vi "Waka manual control.vi"() -> ()   [LabVIEW 2024]
uses:
  ZeroJet Test Systems/Production Data/Production Data.lvlib
  <instrlib>/KDI Digital Instrumentation/API_for_PCAN_BASIC_FD/TPCANBaudrate.ctl
  <instrlib>/KDI Digital Instrumentation/API_for_PCAN_BASIC_FD/TPCANHandle.ctl
  ZeroJet Test Systems/Production Data/TestStand Results/MEASUREMENT power spectrum.vi
  <vilib>/Utility/error.llb/DialogType.ctl
  <userlib>/ZeroJet/IT6000C/IT6000C production.lvlib
  <vilib>/platform/TimedLoop/XDataNode/XDataNode.xnode
  <vilib>/Platform/TimedLoop/XDataNode/nitl_modes.ctl
  <vilib>/Platform/TimedLoop/XDataNode/XDNodeRunTimeDep.lvlib
  <vilib>/Platform/TimedLoop/XDataNode/wakeup.ctl
  <vilib>/Platform/TimedLoop/XDataNode/timing_clust.ctl
  ZeroJet Test Systems/Production Data/TestStand Results/MEASUREMENT float.vi
  ZeroJet Test Systems/Instruments/PCAN/PCan_Xnet.lvlib
  <instrlib>/IT6000C/IT6000C.lvlib
  <vilib>/Utility/sysdir.llb/System Directory Type.ctl
  Helper/Key CAN statistics.ctl
panel:
  in  "stop":bool
  out "Main selector":enum32{"Power supply Setup", "CAN Setup", "Run"}(tab)
  in  "IT6000C instrument address":refnum<visa-resource-name>="USB0::0x2EC7::0x6000::804050011767650001::INSTR"
  in  "Voltage rise time":dbl=5.0 format="%#_13gs"
  in  "Power supply watchdog time":dbl=2.0 min=0.0 max=10.0 step=0.1 format="%#_13gs"
  in  "Button - Connect power supply":bool
  in  "Button - Don't use power supply":bool
  out "LED - Supply connected":bool
  out "Connection response":string
  in  "Button - Power supply next":bool
  in  "Button - Power supply next":bool
  out "LED - Setting up CAN":bool
  out "CAN Status":string
  in  "Vibration capture time (s)":dbl=60.0
  in  "Batch Serial Number":string="RevC Pilot Run"
  in  "Part Number":string="RevC Jet Pump"
  in  "Serial Number":string
  in  "Button - Reset hour counter":bool
  out "Left spectrum channel":cluster{"f0":dbl, "df":dbl, "magnitude":dbl[]}(graph)
  out "Right spectrum channel":cluster{"f0":dbl, "df":dbl, "magnitude":dbl[]}(graph)
  in  "Run tab data":enum32{"Key Data", "All can data", "Errors"}(tab)
  out "Supply wattage output":dbl format="%.2g"
  in  "Current setpoint":dbl(knob) min=0.0 scale=0.06..300.0
  in  "Supply output state":bool
  out "Supply voltage output":dbl format="%.2g"
  out "Supply current output":dbl format="%.2g"
  in  "Voltage setpoint":dbl(knob) min=0.0 scale=0.06..60.0
  out "Key statistics":T1
  out "Signal map":map{string, dbl}(c390)
  out "Error and warning map":map{string, i8}(c390)
  out "Can data write loop":errorcluster
  out "Power supply update loop":errorcluster
  out "Setup loop":errorcluster
  out "Spectrum loop":errorcluster
  # "Power supply setup"
  # "1. Click in this box and select the instrument address for the power supply\n\n\n\n2. Choose the voltage rise time and the watchdog time\n    - Default: 5s votlage rise time\n    - Default: 2s power supply watchdog time\nYou will likely not need to modify these numbers\n\n\n3. Click on connect or don't use power supply\n    - If you are using a battery, then select don't use"
  # "UUT Details"
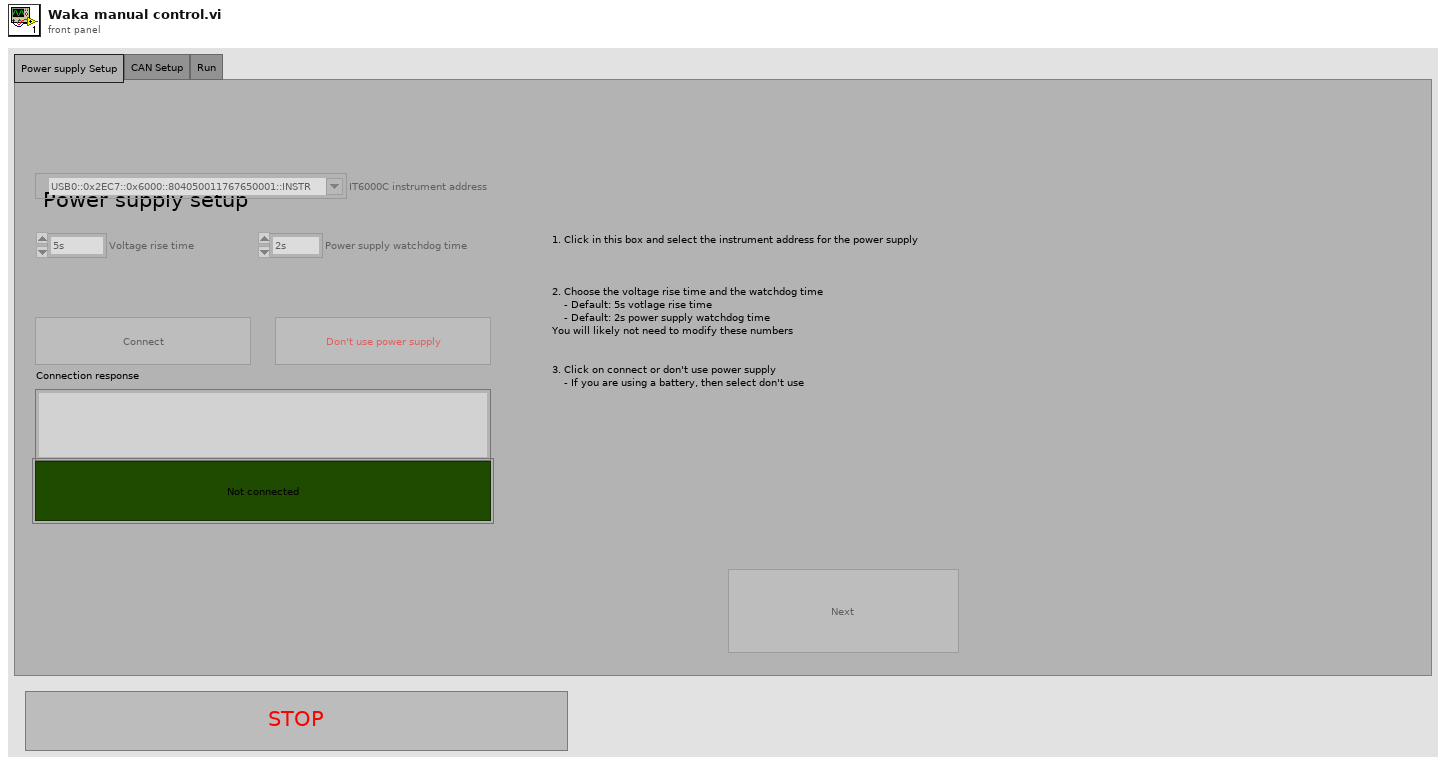
[diagram p1: front panel]
types:
  T1 = typedef "Key CAN statistics.ctl" = cluster{"Drive voltage ":dbl, "High current volt drop":dbl, "High current series resistance":dbl, "Drive phase amps":dbl, "Torque request":dbl, "Motor temp":dbl, "GPS Status":dbl, "RPM":dbl, "Capacitor temp":dbl, "MCM ID":dbl, "MCM Version":string}
  T2 = enum8{"Enabled", "Disabled", "Disabled and Grayed Out"}
  T3 = typedef "TPCANBaudrate.ctl" = enum16{"PCAN_BAUD_1M 0x0014", "PCAN_BAUD_800K 0x0016", "PCAN_BAUD_500K 0x001C", "PCAN_BAUD_250K 0x011C", "PCAN_BAUD_125K 0x031C", "PCAN_BAUD_100K 0x432F", "PCAN_BAUD_95K 0xC34E", "PCAN_BAUD_83K 0x852B", "PCAN_BAUD_50K 0x472F", "PCAN_BAUD_47K 0x1414", "PCAN_BAUD_33K 0x8B2F", "PCAN_BAUD_20K 0x532F", "PCAN_BAUD_10K 0x672F", "PCAN_BAUD_5K 0x7F7F", "User Baudrate"}
  T4 = typedef "TPCANHandle.ctl" = enum16{"PCAN_NONEBUS  0x000", "PCAN_ISABUS1  0x21", "PCAN_ISABUS2  0x22", "PCAN_ISABUS3  0x23", "PCAN_ISABUS4  0x24", "PCAN_ISABUS5  0x25", "PCAN_ISABUS6  0x26", "PCAN_ISABUS7  0x27", "PCAN_ISABUS8  0x28", "PCAN_DNGBUS1  0x31", "PCAN_PCIBUS1  0x41", "PCAN_PCIBUS1  0x42", "PCAN_PCIBUS1  0x43", "PCAN_PCIBUS1  0x44", "PCAN_PCIBUS1  0x45", "PCAN_PCIBUS1  0x46", "PCAN_PCIBUS1  0x47", "PCAN_PCIBUS1  0x48", "PCAN_PCIBUS1  0x409", "PCAN_PCIBUS1  0x40A", "PCAN_PCIBUS1  0x40B", "PCAN_PCIBUS1  0x40C", "PCAN_PCIBUS1  0x40D", "PCAN_PCIBUS1  0x40E", "PCAN_PCIBUS1  0x40F", "PCAN_PCIBUS1  0x410", "PCAN_USBBUS1  0x51", "PCAN_USBBUS2  0x52", "PCAN_USBBUS3  0x53", "PCAN_USBBUS4  0x54", "PCAN_USBBUS5  0x55", "PCAN_USBBUS6  0x56", "PCAN_USBBUS7  0x57", "PCAN_USBBUS8  0x58", "PCAN_USBBUS9  0x509", "PCAN_USBBUS10  0x50A", "PCAN_USBBUS11  0x50B", "PCAN_USBBUS12  0x50C", "PCAN_USBBUS13  0x50D", "PCAN_USBBUS14  0x50E", "PCAN_USBBUS15  0x50F", "PCAN_USBBUS16  0x510", "PCAN_PCCBUS1  0x61", "PCAN_PCCBUS2  0x62", "PCAN_LANBUS1  0x801", "PCAN_LANBUS2  0x802", "PCAN_LANBUS3  0x803", "PCAN_LANBUS4  0x804", "PCAN_LANBUS5  0x805", "PCAN_LANBUS6  0x806", "PCAN_LANBUS7  0x807", "PCAN_LANBUS8  0x808", "PCAN_LANBUS9  0x809", "PCAN_LANBUS10  0x80A", "PCAN_LANBUS11  0x80B", "PCAN_LANBUS12  0x80C", "PCAN_LANBUS13  0x80D", "PCAN_LANBUS14  0x80E", "PCAN_LANBUS15  0x80F", "PCAN_LANBUS16  0x810"}
  T5 = typedef "DialogType.ctl" = u16
  T6 = typedef "NI_Database_API.lvlib/Conn ObjectReference.ctl" = refnum<k1>
  T7 = typedef "System Directory Type.ctl" = i32
  T8 = enum16{"open", "open or create", "create or replace", "create", "open (read-only)"}
  T9 = typedef "XDNodeRunTimeDep.lvlib/timing_clust.ctl" = cluster{"Expected End [f-1]":u64, "Actual End [f-1]":u64, "Finished Late? [f-1]":bool, "Expected End [i-1]":u64, "Actual End [i-1]":u64, "Finished Late? [i-1]":bool, "Expected Start [i]":u64, "Actual Start [i]":u64, "Expected Start [f]":u64, "Actual Start [f]":u64, "Source Name":string, "Structure Name":string, "Period":i64, "Deadline":i64, "Offset":i64, "Start":i64, "Priority":i32, "Timeout":i32, "Mode":T10, "Wakeup Reason":T11, "Error":errorcluster, "Source Type":string, "Secondary Source Type":string, "Global End Time":u64, "Global Start Time":u64, "Frame Duration":u64, "Iteration Duration":u64, "Assigned CPU":i32, "I/O Scan Engine Mode":u32}
  T10 = typedef "XDNodeRunTimeDep.lvlib/nitl_modes.ctl" = enum32{"No Change", "Process missed periods, maintain original phase", "Discard missed periods, maintain original phase", "Process missed periods, ignore original phase", "Discard missed periods, ignore original phase"}
  T11 = typedef "XDNodeRunTimeDep.lvlib/wakeup.ctl" = enum32{"Normal", "Aborted", "Asynchronous wakeup", "Timing source error", "Timed loop error", "Timeout"}
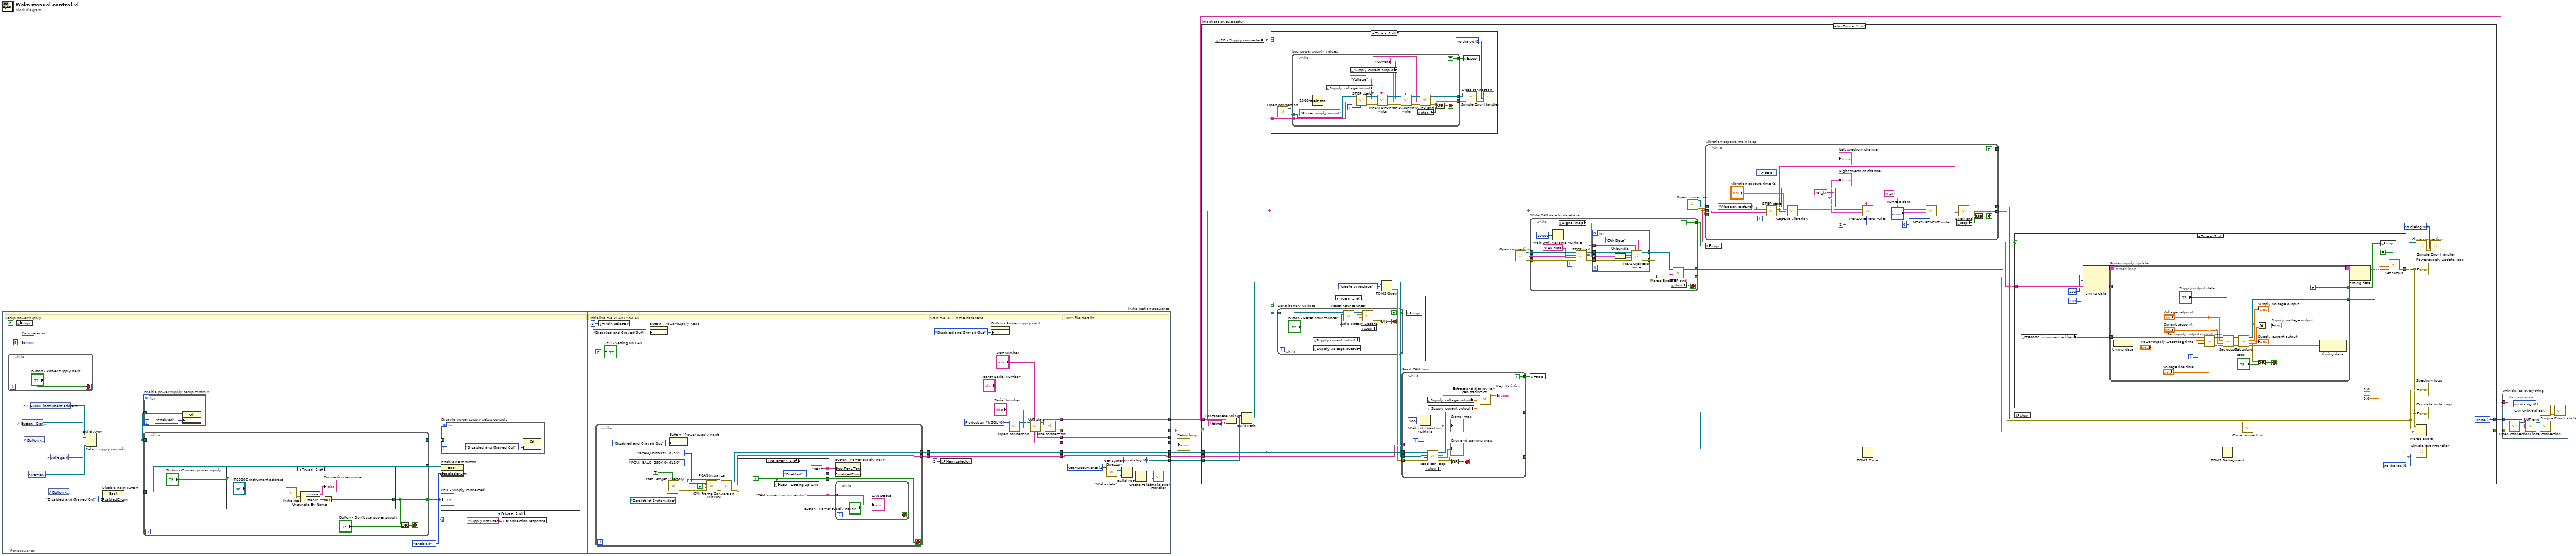
[diagram p0: block diagram]
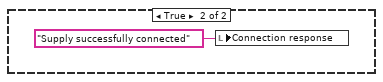
[diagram p2: hidden frame]
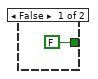
[diagram p3: hidden frame]
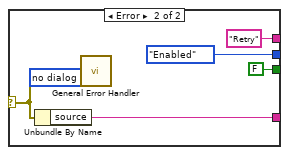
[diagram p4: hidden frame]
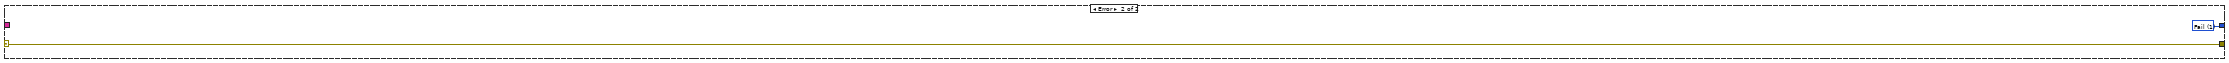
[diagram p8: hidden frame]
diagram:
  n1 = flat-sequence "Initialization sequence" {
    tunnel: [w52] -> w13
    tunnel: [w51] -> w12
    tunnel: w13 -> [w85]
    tunnel: w12 -> [w84]
    tunnel: [w98] -> w9
    tunnel: [w97] -> w8
    tunnel: [w96] -> w7
    tunnel: [w88] -> w6
    tunnel: [w85] -> w5
    tunnel: [w84] -> w4
    tunnel: [w107] -> w10
    tunnel: [w108] -> w11
    tunnel: [w101] -> w2
    tunnel: [w109] -> _
    tunnel: [w110] -> _
    tunnel: [w111] -> w15
    tunnel: w9 -> [w111]
    tunnel: w8 -> [w110]
    tunnel: w7 -> [w109]
    tunnel: w6 -> [w101]
    tunnel: w5 -> [w108]
    tunnel: w4 -> [w107]
    tunnel: [w103] -> w3
    frame #0 {
      # "Setup power supply"
      n2 = while {
        stop <- "Button - Power supply next" stop-if-true
      }
      n3 = local write "stop"(FALSE ("Release all channels first")) -> ()
      n4 = control-ref of="Button - Don't use power supply"() -> (w29:refnum<vi>)
      n5 = control-ref of="Button - Connect power supply"() -> (w28:refnum<vi>)
      n6 = control-ref of="Power supply watchdog time"() -> (w26:refnum<vi>)
      n7 = control-ref of="IT6000C instrument address"() -> (w30:refnum<vi>)
      n8 = control-ref of="Button - Power supply next"() -> (w22:refnum<vi>)
      n9 = control-ref of="Voltage rise time"() -> (w27:refnum<vi>)
      n10 = Build Array "Select supply controls"(w30, w29, w28, w27, w26) -> (w24:refnum<vi>[])
      n11 = property on="Disable next button" class="Bool"(reference=w22, "DisabledEnum"=T2."Disabled and Grayed Out" ("Disabled")) -> (reference out=w19:refnum<vi>)  [unwired: 1 in, 1 out]
      n12 = for "Enable power supply setup controls" {
        tunnel: w24 -> [w34] mode=indexing
        n13 = property class="Ctl"(reference=w34, "DisabledEnum"=T2."Enabled" ("Disabled")) -> ()  [unwired: 1 in, 2 out]
      }
      n14 = while {
        tunnel: [w40] -> w17
        tunnel: [w39] -> w25
        tunnel: w24 -> [w39]
        tunnel: [w38] -> w20
        tunnel: w19 -> [w38]
        stop <- w41 stop-if-true
        n15 = case shown="True" "Button - Connect power supply" {
          tunnel: [FALSE w46] -> w40
          frame False {
          }
          frame True {
            n16 = call <instrlib>:"Initialize.vi"("VISA resource name"="IT6000C instrument address") -> ("error out"=w48:errorcluster)  [unwired: 9 in, 1 out]
            n17 = Unbundle By Name(w48) -> ("source"=→"Connection response":string, "status"=w47:bool)
            n18 = Not(x=w47) -> (.not. x?=w46:bool)
          }
        }
        n19 = Or(x=w40, y="Button - Don't use power supply") -> (x .or. y?=w41:bool)
      }
      "LED - Supply connected" <- w17
      n20 = for "Disable power supply setup controls" {
        tunnel: w25 -> [w32] mode=indexing
        n21 = property class="Ctl"(reference=w32, "DisabledEnum"=T2."Disabled and Grayed Out" ("Disabled")) -> ()  [unwired: 1 in, 2 out]
      }
      n22 = property on="Enable next button" class="Bool"(reference=w20, "DisabledEnum"=T2."Enabled" ("Disabled")) -> ()  [unwired: 1 in, 2 out]
      n23 = case "Update connection response" shown="False" w17 {
        frame False {
          n24 = local write "Connection response"("Supply not used" ("Connection response")) -> ()
        }
        frame True {
          n25 = local write "Connection response"("Supply successfully connected" ("Connection response")) -> ()
        }
      }
      "Main selector" <- 0
    }
    frame #1 {
      # "Initialise the PCAN USB-CAN"
      n26 = while {
        tunnel: [w66] -> w51
        tunnel: [w65] -> w52
        stop <- w57 stop-if-true
        n27 = call "Get ZeroJet Directory.vi"("Expect file to be present"=TRUE, "Data directory subpath"=path "ZeroJet Jet System.dbc") -> ("error out"=w62:errorcluster, "appended path"=w63:path)  [unwired: 7 in, 1 out]
        n28 = property on="Button - Power supply next" class="Bool"("DisabledEnum"=T2."Disabled and Grayed Out" ("Disabled")) -> ()  [unwired: 2 in, 2 out]
        n29 = call "PCAN Initialize.vi"("error in"=w62, "Release all channels first"=TRUE, "TPCANBaudrate"=TPCANBaudrate."PCAN_BAUD_250K 0x011C", "TPCANHandle"=TPCANHandle."PCAN_USBBUS1  0x51") -> ("error out"=w67:errorcluster)  [unwired: 6 in, 1 out]
        n30 = call "CAN Frame Conversion - Init DBC.vi"("error in (no error)"=w67, "DBC Path"=w63) -> ("error out"=w61:errorcluster, "Signals For Conversion"=w66:string[], "Frame Signal Conversion out"=w65:refnum<class "Frame Signal Conversion.lvclass">)  [unwired: 7 in]
        n31 = case shown="No Error" w61 {
          selector: w61 -> [_ w76]
          tunnel: ["Next" ("Boolean Text.Text") "Retry" ("Boolean Text.Text")] -> w59
          tunnel: [T2."Enabled" ("Disabled") T2."Enabled" ("Disabled")] -> w58
          tunnel: ["CAN connection successful" ("source") w78] -> w56
          tunnel: [w71 FALSE ("LED - Setting up CAN")] -> w57
          frame No Error {
            w71 = TRUE ("LED - Setting up CAN")
            n32 = local write "LED - Setting up CAN"(w71) -> ()
          }
          frame Error {
            w75 = T5 0 items=["no dialog", "OK message", "continue or stop message", "OK message + warnings", "continue/stop + warnings"] ("type of dialog (OK msg:1)")
            n33 = Unbundle By Name(w76) -> ("source"=w78:string)
            n34 = call <vilib>:"General Error Handler.vi"("type of dialog (OK msg:1)"=w75, "error in (no error)"=w76) -> ()  [unwired: 9 in, 5 out]
          }
        }
        n35 = property on="Button - Power supply next" class="Bool"("BoolText.Text"=w59, "DisabledEnum"=w58) -> ()  [unwired: 2 in, 2 out]
        n36 = while {
          tunnel: w56 -> [w81]
          stop <- "Button - Power supply next" stop-if-true
          "CAN Status" <- w81
        }
      }
      n37 = local write "Main selector"(1) -> ()
      n38 = property on="Button - Power supply next" class="Bool"("DisabledEnum"=T2."Disabled and Grayed Out" ("Disabled")) -> ()  [unwired: 2 in, 2 out]
      "LED - Setting up CAN" <- FALSE
    }
    frame #2 {
      w87 = u16 0 items=["Production MySQL"] ("Database")
      # "Start the UUT in the database"
      n39 = local write "Main selector"(2) -> ()
      n40 = property on="Button - Power supply next" class="Bool"("DisabledEnum"=T2."Disabled and Grayed Out" ("Disabled")) -> ()  [unwired: 2 in, 2 out]
      n41 = call "Open connection.vi"("Database"=w87) -> ("error out"=w91:errorcluster, "connection reference"=w93:T6)  [unwired: 9 in]
      n42 = call "UUT start.vi"("Part Number"="Part Number", "error in (no error)"=w91, "Serial Number"="Serial Number", "Batch Serial Number"="Batch Serial Number", "connection reference"=w93) -> ("error out"=w89:errorcluster, "UUT GUID"=w98:string, "connection reference out"=w90:T6, "Username"=w97:string, "Station name"=w96:string)  [unwired: 2 in]
      n43 = call "Close connection.vi"("error in"=w89, "connection reference"=w90) -> ("error out"=w88:errorcluster)  [unwired: 9 in]
    }
    frame #3 {
      w102 = T7 2 items=["User Home"=0, "User Desktop"=1, "User Documents"=2, "User Application Data"=3, "User Preferences"=4, "User Temporary"=5, "Public Documents"=6, "Public Application Data"=7, "Public Preferences"=8, "Public Cache"=13, "System Core Libraries"=9, "System Installed Libraries"=10, "Application Files"=11, "Boot Volume Root"=12] ("system directory type")
      w99 = T5 0 items=["no dialog", "OK message", "continue or stop message", "OK message + warnings", "continue/stop + warnings"] ("type of dialog (OK msg:1)")
      # "TDMS file details"
      n44 = call <vilib>:"Get System Directory.vi"("system directory type"=w102) -> ("system directory"=w106:path)  [unwired: 10 in]
      n45 = Build Path(base path=w106, name or relative path=path "Waka data") -> (appended path=w104:path)
      n46 = Create Folder(path (use dialog)=w104) -> (created path=w103:path, error out=w100:errorcluster)  [unwired: 2 in, 1 out]
      n47 = call <vilib>:"Simple Error Handler.vi"("type of dialog (OK msg:1)"=w99, "error in (no error)"=w100) -> ()  [unwired: 3 in, 5 out]
    }
  }
  n48 = case "Initialization successful" shown="No Error" w2 {
    selector: w2 -> [_ w294]
    tunnel: w15 -> [w142 _]
    tunnel: [w145 w295] -> w14
    tunnel: w11 -> [w140 _]
    tunnel: w10 -> [w139 _]
    tunnel: w3 -> [w141 _]
    tunnel: [w117 w294] -> w1
    frame No Error {
      w132 = T5 0 items=["no dialog", "OK message", "continue or stop message", "OK message + warnings", "continue/stop + warnings"] ("type of dialog (OK msg:1)")
      w135 = T5 0 items=["no dialog", "OK message", "continue or stop message", "OK message + warnings", "continue/stop + warnings"] ("type of dialog (OK msg:1)")
      w145 = u16 2 items=["Pass", "Fail", "Done", "Error"] ("Test Result")
      n49 = local read "LED - Supply connected"() -> (w112:bool)
      n50 = Concatenate Strings(w142, ".tdms" ("string")) -> (w120:string)
      n51 = Build Path(base path=w141, name or relative path=w120) -> (appended path=w119:path)
      n52 = case shown="True" w112 {
        tunnel: w142 -> [_ w149]
        frame False {
        }
        frame True {
          w148 = T5 0 items=["no dialog", "OK message", "continue or stop message", "OK message + warnings", "continue/stop + warnings"] ("type of dialog (OK msg:1)")
          n53 = call "Open connection.vi"() -> ("connection reference"=w147:T6)  [unwired: 10 in, 1 out]
          n54 = while "Log power supply values" {
            tunnel: w147 -> [w173]
            tunnel: w149 -> [w165]
            tunnel: [w158] -> w146
            tunnel: [w154] -> w150
            tunnel: [TRUE] -> w152
            i -> [w156]
            stop <- w159 stop-if-true
            n55 = Wait (ms)(milliseconds to wait=u32 1000) -> ()  [unwired: 1 out]
            n56 = local read "Supply voltage output"() -> (w168:dbl)
            n57 = local read "Supply current output"() -> (w169:dbl)
            n58 = call "STEP start.vi"("Loop index"=w156, "UUT GUID"=w165, "Step name"="Power supply output" ("Step category"), "connection reference"=w173) -> ("error out"=w163:errorcluster, "Step GUID"=w164:string, "connection reference out"=w172:T6)  [unwired: 5 in]
            n59 = call-poly "MEASUREMENT write.vi"("Step Parent GUID"=w164, "error in (no error)"=w163, "Input data"=w168, "Step name"="Voltage", "connection reference"=w172) -> ("error out"=w162:errorcluster, "connection reference out"=w171:T6)  [unwired: 4 in, 1 out]
            n60 = call-poly "MEASUREMENT write.vi"("Step Parent GUID"=w164, "error in (no error)"=w162, "Input data"=w169, "Step name"="Current", "connection reference"=w171) -> ("error out"=w161:errorcluster, "connection reference out"=w170:T6)  [unwired: 4 in, 1 out]
            n61 = local read "stop"() -> (w160:bool)
            n62 = call "STEP end.vi"("error in (no error)"=w161, "Step GUID"=w164, "connection reference"=w170) -> ("error out"=w158:errorcluster, "connection reference out"=w154:T6)  [unwired: 7 in]
            n63 = Or(x=w158, y=w160) -> (x .or. y?=w159:bool)
          }
          n64 = local write "stop"(w152) -> ()
          n65 = call "Close connection.vi"("error in"=w146, "connection reference"=w150) -> ("error out"=w151:errorcluster)  [unwired: 9 in]
          n66 = call <vilib>:"Simple Error Handler.vi"("type of dialog (OK msg:1)"=w148, "error in (no error)"=w151) -> ()  [unwired: 3 in, 5 out]
        }
      }
      n67 = case shown="True" w112 {
        tunnel: w140 -> [_ w175]
        frame False {
        }
        frame True {
          n68 = while "Send battery update" {
            tunnel: w175 -> [w177]
            tunnel: [TRUE] -> w174
            stop <- w183 stop-if-true
            n69 = local read "Supply current output"() -> (w180:dbl)
            n70 = local read "Supply voltage output"() -> (w179:dbl)
            n71 = call "Reset hour counter.vi"("Button - Reset hour counter"="Button - Reset hour counter", "Frame Signal Conversion in"=w177) -> ("Frame Signal Conversion out"=w176:refnum<class "Frame Signal Conversion.lvclass">)  [unwired: 8 in, 1 out]
            n72 = local read "stop"() -> (w184:bool)
            n73 = call "Waka battery update.vi"("Supply Voltage"=w179, "Supply Current"=w180, "Frame Signal Conversion in"=w176) -> ("error out"=w182:errorcluster)  [unwired: 8 in]
            n74 = Or(x=w182, y=w184) -> (x .or. y?=w183:bool)
          }
          n75 = local write "stop"(w174) -> ()
        }
      }
      n76 = TDMS Open(10:T8."create or replace" ("operation (0:open)"), 11:w119) -> (0:w134:errorcluster, 3:w133:refnum<k34>)  [unwired: 5 in]
      n77 = while "Read CAN loop" {
        tunnel: w140 -> [w226]
        tunnel: w139 -> [w225]
        tunnel: [w220] -> w118
        tunnel: [TRUE ("stop")] -> w128
        tunnel: w134 -> [w222]
        tunnel: w133 -> [w221]
        tunnel: [w219] -> w131
        i -> [w217]
        stop <- w223 stop-if-true
        n78 = Wait Until Next ms Multiple(millisecond multiple=u32 100) -> ()  [unwired: 1 out]
        n79 = local read "stop"() -> (w218:bool)
        n80 = local read "Supply voltage output"() -> (w215:dbl)
        n81 = call "Read can loop.vi"("Signals For Conversion"=w225, "error in (no error)"=w222, "Numeric"=w217, "tdms file in"=w221, "Frame Signal Conversion in"=w226) -> ("error out"=w220:errorcluster, "Error and warning map"=→"Error and warning map":map{string, i8}, "Signal map"=w212:map{string, dbl}, "tdms file out"=w219:refnum<k34>)  [unwired: 3 in]
        "Signal map" <- w212
        n82 = local read "Supply current output"() -> (w214:dbl)
        n83 = Or(x=w220, y=w218) -> (x .or. y?=w223:bool)
        n84 = call "Extract and display key can statisctics.vi"("Supply current output"=w214, "Supply voltage output"=w215, "Signal map in"=w212) -> ("Key statistics"=→"Key statistics":T1)  [unwired: 8 in]
      }
      n85 = call "Open connection.vi"() -> ("error out"=w124:errorcluster, "connection reference"=w126:T6)  [unwired: 10 in]
      n86 = while "Write CAN data to database" {
        tunnel: [TRUE] -> w127
        tunnel: w126 -> [w195]
        tunnel: [w194] -> w125
        tunnel: w124 -> [w193]
        tunnel: [w189] -> w123
        tunnel: w142 -> [w186]
        i -> [w185]
        stop <- w200 stop-if-true
        n87 = Wait Until Next ms Multiple(millisecond multiple=u32 10000) -> ()  [unwired: 1 out]
        n88 = local read "Signal map"() -> (w196:map{string, dbl})
        n89 = call "STEP start.vi"("Loop index"=w185, "error in (no error)"=w193, "UUT GUID"=w186, "Step name"="CAN data", "connection reference"=w195) -> ("error out"=w192:errorcluster, "Step GUID"=w188:string, "connection reference out"=w198:T6)  [unwired: 4 in]
        n90 = for {
          tunnel: w198 -> [w210]
          tunnel: [w209] -> w197
          tunnel: w196 -> [w208] mode=indexing
          tunnel: w188 -> [w205]
          tunnel: w192 -> [w203]
          tunnel: [w202] -> w191 mode=indexing
          n91 = Unbundle(w208) -> (w207:string, w206:dbl)
          n92 = call-poly "MEASUREMENT write.vi"("Step category"="CAN Data", "Step Parent GUID"=w205, "error in (no error)"=w203, "Input data"=w206, "Step name"=w207, "connection reference"=w210) -> ("error out"=w202:errorcluster, "connection reference out"=w209:T6)  [unwired: 3 in, 1 out]
        }
        n93 = Merge Errors(w191) -> (w190:errorcluster)
        n94 = local read "stop"() -> (w200:bool)
        n95 = call "STEP end.vi"("error in (no error)"=w190, "Step GUID"=w188, "connection reference"=w197) -> ("error out"=w189:errorcluster, "connection reference out"=w194:T6)  [unwired: 7 in]
      }
      n96 = local write "stop"(w128) -> ()
      n97 = call "Open connection.vi"() -> ("error out"=w137:errorcluster, "connection reference"=w138:T6)  [unwired: 10 in]
      n98 = while "Vibration capture main loop" {
        tunnel: w142 -> [w247]
        tunnel: [w237] -> w144
        tunnel: [w230] -> w114
        tunnel: [TRUE] -> w143
        tunnel: w138 -> [w228]
        tunnel: w137 -> [w227]
        i -> [w236]
        stop <- w250 stop-if-true
        n99 = control-ref of="stop"() -> ()  [unwired: 1 out]
        n100 = call "STEP start.vi"("Loop index"=w236, "error in (no error)"=w227, "UUT GUID"=w247, "Step name"="Vibration capture", "connection reference"=w228) -> ("error out"=w246:errorcluster, "Step GUID"=w239:string, "connection reference out"=w245:T6)  [unwired: 4 in]
        n101 = call "Capture vibration.vi"("error in (no error)"=w246, "Vibration capture time (s)"="Vibration capture time (s)") -> ("error out"=w231:errorcluster, "Frequency power spectrum"=w232:cluster{"f0":dbl, "df":dbl, "magnitude":dbl[]}, "Frequency power spectrum 2"=w233:cluster{"f0":dbl, "df":dbl, "magnitude":dbl[]})  [unwired: 7 in]
        "Left spectrum channel" <- w233
        "Right spectrum channel" <- w232
        n102 = call-poly "MEASUREMENT write.vi"("Order number"=1, "Step GUID"=w239, "error in (no error)"=w231, "Input frequency power spectrum"=w232, "Step name"="Right", "connection reference"=w245) -> ("error out"=w244:errorcluster, "connection reference out"=w243:T6)  [unwired: 3 in, 1 out]
        n103 = call-poly "MEASUREMENT write.vi"("Order number"=0, "Step GUID"=w239, "error in (no error)"=w244, "Input frequency power spectrum"=w233, "Step name"="Left", "connection reference"=w243) -> ("error out"=w240:errorcluster, "connection reference out"=w238:T6)  [unwired: 3 in, 1 out]
        n104 = local read "stop"() -> (w249:bool)
        n105 = call "STEP end.vi"("error in (no error)"=w240, "Step GUID"=w239, "connection reference"=w238) -> ("error out"=w230:errorcluster, "connection reference out"=w237:T6)  [unwired: 7 in]
        n106 = Or(x=w230, y=w249) -> (x .or. y?=w250:bool)
      }
      "Spectrum loop" <- w114
      n107 = local write "stop"(w127) -> ()
      n108 = TDMS Close(8:w118, 11:w131) -> (0:w129:errorcluster, 3:w130:path)
      n109 = case shown="True" w112 {
        tunnel: w142 -> [_ w264]
        tunnel: [_ w253] -> w113
        frame False {
        }
        frame True {
          n110 = local read "IT6000C instrument address"() -> (w252:refnum<visa-resource-name>)
          n111 = node-c288(i64 100 ("Period"), 100 ("Priority")) -> (w258:T9)  [unwired: 1 in]
          n112 = timed-loop "Power supply update" {
            tunnel: w264 -> [_]
            tunnel: [TRUE] -> w254
            timing: w258 -> [_]
            timing-out: [_] -> w257
            tunnel: [w282] -> w260
            tunnel: w252 -> [w273]
            i -> [w276]
            stop <- w280 stop-if-true
            n113 = node-c288() -> ()  [unwired: 1 in]
            n114 = call "Set supply output on first loop.vi"("Current"="Current setpoint", "Voltage rise time"="Voltage rise time", "Voltage"="Voltage setpoint", "Numeric"=w276, "Power supply watchdog time"="Power supply watchdog time", "VISA Refnum in"=w273) -> ("error out"=w269:errorcluster, "VISA Refnum out"=w272:refnum<visa-resource-name>)  [unwired: 4 in]
            n115 = call <userlib>:"Set output.vi"("Output state"="Supply output state", "error in"=w269, "Current(A)"="Current setpoint", "Voltage(V)"="Voltage setpoint", "VISA resource name"=w272) -> ("error out"=w277:errorcluster, "VISA resource name out"=w278:refnum<visa-resource-name>)  [unwired: 5 in]
            n116 = call <userlib>:"Get output.vi"("error in"=w277, "VISA resource name"=w278) -> ("error out"=w281:errorcluster, "Actual Current Level (A)"=w266:dbl, "Actual Voltage Level (V)"=w267:dbl, "VISA resource name out"=w282:refnum<visa-resource-name>)  [unwired: 6 in]
            "Supply current output" <- w266
            "Supply voltage output" <- w267
            n117 = Or(x=w281, y="stop") -> (x .or. y?=w280:bool)
            n118 = Multiply(x=w267, y=w266) -> (x*y=→"Supply wattage output":dbl)
            n119 = node-c288(w281) -> ()  [unwired: 1 out]
          }
          n120 = node-c288(w257) -> (w259:errorcluster)
          n121 = local write "stop"(w254) -> ()
          n122 = call <userlib>:"Set output.vi"("Output state"=FALSE, "error in"=w259, "Current(A)"=0.0, "Voltage(V)"=0.0, "VISA resource name"=w260) -> ("error out"=w253:errorcluster)  [unwired: 5 in, 1 out]
        }
      }
      "Power supply update loop" <- w113
      n123 = local write "stop"(w143) -> ()
      n124 = TDMS Defragment(4:w129, 7:w130) -> (0:w116:errorcluster)
      n125 = call "Close connection.vi"("error in"=w123, "connection reference"=w125) -> ("error out"=w115:errorcluster)  [unwired: 9 in]
      "Can data write loop" <- w115
      n126 = call "Close connection.vi"("connection reference"=w144) -> ("error out"=w136:errorcluster)  [unwired: 10 in]
      n127 = Merge Errors(w113, w114, w115, w116) -> (w117:errorcluster)
      n128 = call <vilib>:"Simple Error Handler.vi"("type of dialog (OK msg:1)"=w132, "error in (no error)"=w116) -> ()  [unwired: 3 in, 5 out]
      n129 = call <vilib>:"Simple Error Handler.vi"("type of dialog (OK msg:1)"=w135, "error in (no error)"=w136) -> ()  [unwired: 3 in, 5 out]
    }
    frame Error {
      w295 = u16 1 items=["Pass", "Fail", "Done", "Error"] ("Test Result")
    }
  }
  n130 = flat-sequence "Uninitialize everything" {
    tunnel: w15 -> [w298]
    tunnel: w14 -> [w297]
    tunnel: w1 -> [w296]
    frame #0 {
      w303 = T5 0 items=["no dialog", "OK message", "continue or stop message", "OK message + warnings", "continue/stop + warnings"] ("type of dialog (OK msg:1)")
      n131 = call "Open connection.vi"("error in"=w296) -> ("error out"=w301:errorcluster, "connection reference"=w302:T6)  [unwired: 9 in]
      n132 = call "UUT end.vi"("error in (no error)"=w301, "Test UUID"=w298, "Test Result"=w297, "connection reference"=w302) -> ("error out"=w299:errorcluster, "connection reference out"=w300:T6)  [unwired: 6 in]
      n133 = call <instrlib>:"CAN Uninitialize.vi"() -> ("error out"=w304:errorcluster)  [unwired: 9 in, 2 out]
      n134 = call "Close connection.vi"("error in"=w299, "connection reference"=w300) -> ()  [unwired: 9 in, 1 out]
      n135 = call <vilib>:"Simple Error Handler.vi"("type of dialog (OK msg:1)"=w303, "error in (no error)"=w304) -> ()  [unwired: 3 in, 5 out]
    }
  }
  "Setup loop" <- w2
